vi "Configuration Error Info.vi"(11 "configuration error":T1(ring)) -> (3 "error info":cluster{"code":i32, "description":string})   [LabVIEW 2017, in "DSF Core.lvlib" / "Configuration Session.lvclass"]
uses:
  Configuration Session.lvclass
  Shared/Constants/Base Error Code.vi
  Shared/Constants/Error Offset (Configuration).vi
  DSF Core.lvlib
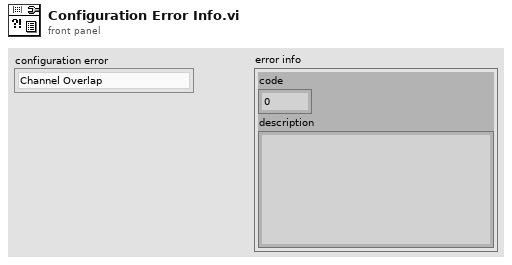
[diagram p1: front panel]
types:
  T1 = enum16{"Channel Overlap", "Invalid Engine Offset"}
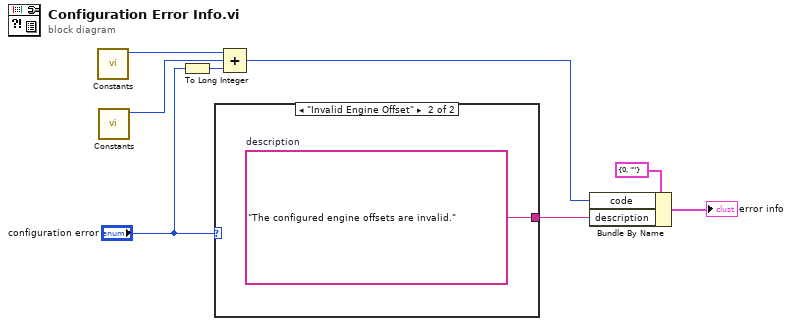
[diagram p0: block diagram]
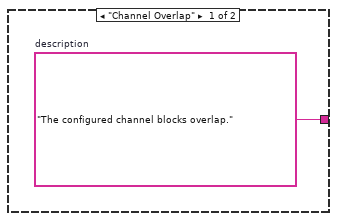
[diagram p2: hidden frame]
diagram:
  n1 = call-poly "Constants.vi"() -> ("base error code"=w7:i32)  [unwired: 11 in]
  n2 = call-poly "Constants.vi"() -> ("error code offset"=w8:i32)  [unwired: 11 in]
  n3 = To Long Integer(number="configuration error") -> (32bit integer=w3:i32)
  n4 = case shown="\"Invalid Engine Offset\"" "configuration error" {
    tunnel: [w9 w10] -> w5
    frame "Channel Overlap" {
      w9 = "The configured channel blocks overlap."  # description
    }
    frame "Invalid Engine Offset" {
      w10 = "The configured engine offsets are invalid."  # description
    }
  }
  n5 = Compound Arithmetic op=ADD(w7, w8, w3) -> (w1:i32)
  n6 = Bundle By Name(cluster=cluster{"code":i32, "description":string} {"code"=0, "description"=""}, "code"=w1, "description"=w5) -> (→"error info":cluster{"code":i32, "description":string})
